vi "setUp.vi"(8 "error in (no error)":errorcluster, 11 "reference in":refnum<class "Routing and Faulting State Value Table Unit Tests.lvclass">) -> (0 "error out":errorcluster, 3 "reference out":refnum<class "Routing and Faulting State Value Table Unit Tests.lvclass">)   [LabVIEW 2020, in "Routing and Faulting State Value Table Unit Tests.lvclass"]
doc: "setUp runs prior to the test method during test execution. Use this method to initialize any object data required by your tests."
uses:
  Routing and Faulting State Value Table Unit Tests.lvclass
  C:/Program Files (x86)/National Instruments/LabVIEW 2020/vi.lib/addons/_JKI Toolkits/VI Tester/TestCase.llb/TestCase.lvclass
  NationalInstruments.VeriStand.SystemDefinitionAPI
  Routing and Faulting State Value Table Unit Tests.lvclass/Routing and Faulting State Value Table Unit Tests.ctl
  <userlib>/_OpenG.lib/file/file.llb/Append Path to Root if Relative - Scalar__ogtk.vi
  <vilib>/addons/_JKI Toolkits/VI Tester/TestCase.llb/TestCase.lvclass
  <vilib>/NI/VeriStand Custom Device Testing Tools/VeriStandTestUtilities/VeriStandTestUtilities.lvlib
  Scripting/Routing and Faulting Scripting.lvlib
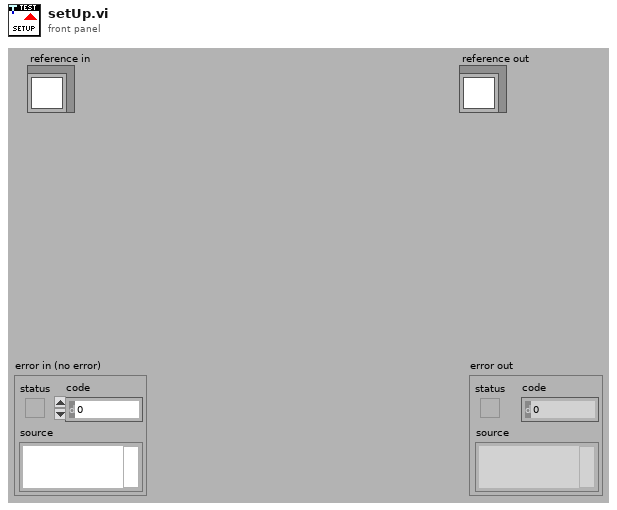
[diagram p1: front panel]
types:
  T1 = typedef "Custom Device API.lvlib/Custom Device Item Ref.ctl" = u64
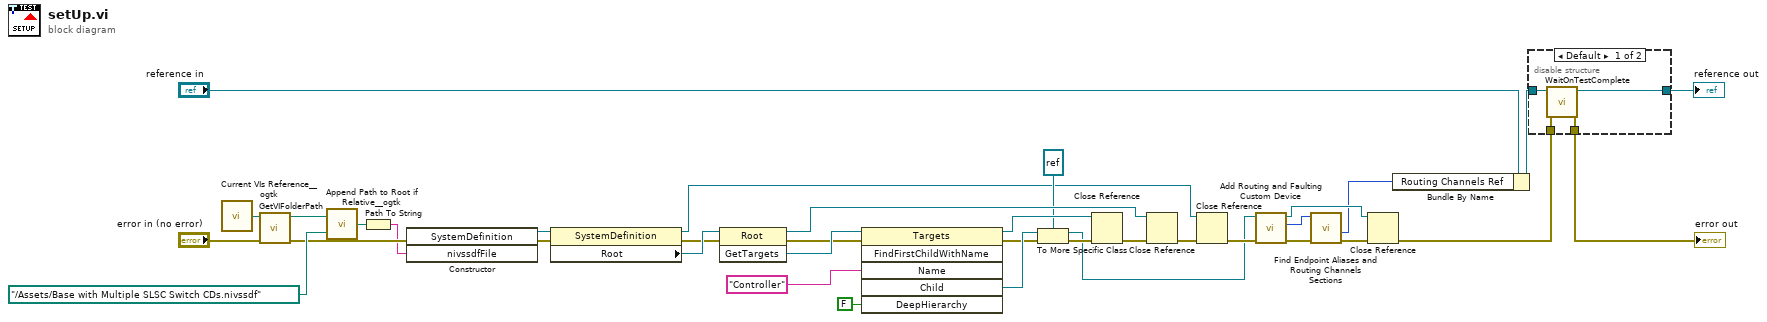
[diagram p0: block diagram]
diagram:
  n1 = call <userlib>:"Current VIs Reference__ogtk.vi"() -> ("Current VI's reference"=w32:refnum<vi>)  [unwired: 5 in]
  n2 = call <vilib>:"GetVIFolderPath.vi"("error in (no error)"="error in (no error)", "VI Reference in"=w32) -> ("error out"=w28:errorcluster, "VI Folder Path out"=w31:path)  [unwired: 8 in]
  n3 = call-poly <userlib>:"Append Path to Root if Relative__ogtk.vi"("Absolute or Relative Path"=path "../Assets/Base with Multiple SLSC Switch CDs.nivssdf", "Root Path"=w31) -> ("Absolute or Appended Path"=w29:path)
  n4 = Path To String(path=w29) -> (string=w27:string)
  n5 = constructor class="SystemDefinition"(error in=w28, "nivssdfFile"=w27) -> (reference out=w12:refnum<k24>, error out=w13:errorcluster)  [unwired: 2 in, 2 out]
  n6 = property class="SystemDefinition"(reference=w12, error in=w13) -> (reference out=w9:refnum<k24>, error out=w22:errorcluster, "Root"=w23:refnum<k24>)
  n7 = invoke class="Root" method="GetTargets"(reference=w23, error in=w22) -> (reference out=w19:refnum<k24>, error out=w24:errorcluster, "GetTargets"=w25:refnum<k24>)  [unwired: 1 in]
  n8 = invoke class="Targets" method="FindFirstChildWithName"(reference=w25, error in=w24, "Name"="Controller", "DeepHierarchy"=FALSE) -> (reference out=w21:refnum<k24>, error out=w16:errorcluster, "Child"=w18:refnum<k24>)  [unwired: 2 in, 3 out]
  n9 = To More Specific Class(target class=refnum<k24> refnum ("reference out"), reference=w18, error in=w16) -> (specific class reference=w7:refnum<k24>, error out=w15:errorcluster)
  n10 = Close Reference(reference=w21, error in (no error)=w15) -> (error out=w20:errorcluster)
  n11 = Close Reference(reference=w19, error in (no error)=w20) -> (error out=w10:errorcluster)
  n12 = Close Reference(reference=w9, error in (no error)=w10) -> (error out=w8:errorcluster)
  n13 = call "Add Routing and Faulting Custom Device.vi"("error in"=w8, "target in"=w7) -> ("error out"=w26:errorcluster, "routing and faulting custom device"=w6:T1, "target out"=w3:refnum<k24>)  [unwired: 7 in]
  n14 = call "Find Endpoint Aliases and Routing Channels Sections.vi"("error in"=w26, "routing and faulting custom device in"=w6) -> ("error out"=w2:errorcluster, "routing channels"=w1:T1)  [unwired: 6 in, 2 out]
  n15 = Close Reference(reference=w3, error in (no error)=w2) -> (error out=w4:errorcluster)
  n16 = Bundle By Name(cluster="reference in", "Routing Channels Ref"=w1) -> (w33:refnum<class "Routing and Faulting State Value Table Unit Tests.lvclass">)
  n17 = disable-structure shown="Default" {
    disable-tunnel: w4 -> [w40 w41]
    disable-tunnel: [w39 w41] -> w36
    disable-tunnel: [w38 w42] -> w34
    disable-tunnel: w33 -> [w37 w42]
    frame condition #0 (active) {
      n18 = call <vilib>:"WaitOnTestComplete.vi"("error in (no error)"=w40, "TestCase in"=w37) -> ("error out"=w39:errorcluster, "TestCase out"=w38:refnum<class "Routing and Faulting State Value Table Unit Tests.lvclass">)  [unwired: 8 in]
    }
    frame condition #1 {
    }
  }
  "error out" <- w36
  "reference out" <- w34
